vi "CheckIfCoordinBox.vi"(10 "axis info":T1, 11 "Box bounds":T2) -> (3 "In Box":bool)   [LabVIEW 2023, in "FolloWin.lvclass"]
doc: "This VI checks if Horizontal and Vertical values of axis info lie within Box bound"
uses:
  FolloWin.lvclass
  <vilib>/Utility/miscctls.llb/LVRectTypeDef.ctl
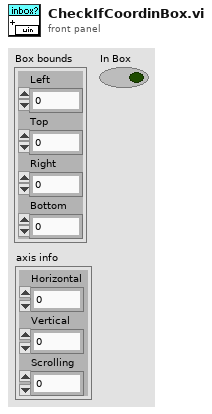
[diagram p1: front panel]
types:
  T1 = cluster{"Horizontal":i32, "Vertical":i32, "Scrolling":i32}
  T2 = typedef "LVRectTypeDef.ctl" = cluster{"Left":i16, "Top":i16, "Right":i16, "Bottom":i16}
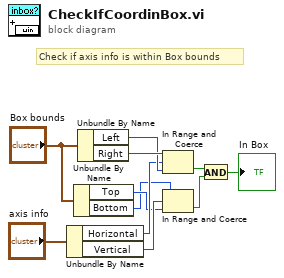
[diagram p0: block diagram]
diagram:
  # "Check if axis info is within Box bounds"
  n1 = Unbundle By Name("axis info") -> ("Horizontal"=w4:i32, "Vertical"=w5:i32)
  n2 = Unbundle By Name("Box bounds") -> ("Top"=w2:i16, "Bottom"=w1:i16)
  n3 = Unbundle By Name("Box bounds") -> ("Left"=w6:i16, "Right"=w7:i16)
  n4 = In Range and Coerce(upper limit=w7, x=w4, lower limit=w6) -> (In Range?=w8:bool)  [unwired: 1 out]
  n5 = In Range and Coerce(upper limit=w1, x=w5, lower limit=w2) -> (In Range?=w9:bool)  [unwired: 1 out]
  n6 = And(x=w8, y=w9) -> (x .and. y?=→"In Box":bool)
